vi "Set Manual Volt per Division.vi"(8 "error in (no error)":errorcluster, 9 "V/div":T1, 11 "Oscilloscope in":refnum<class "Oscilloscope.lvclass">) -> (0 "error out":errorcluster, 3 "Oscilloscope out":refnum<class "Oscilloscope.lvclass">)   [LabVIEW 2018, in "Oscilloscope.lvlib" / "Oscilloscope.lvclass"]
uses:
  Oscilloscope.lvclass
  Custom Controls/Volts per Division.ctl
  Custom Controls/Analog Channels.ctl
  Oscilloscope.lvlib
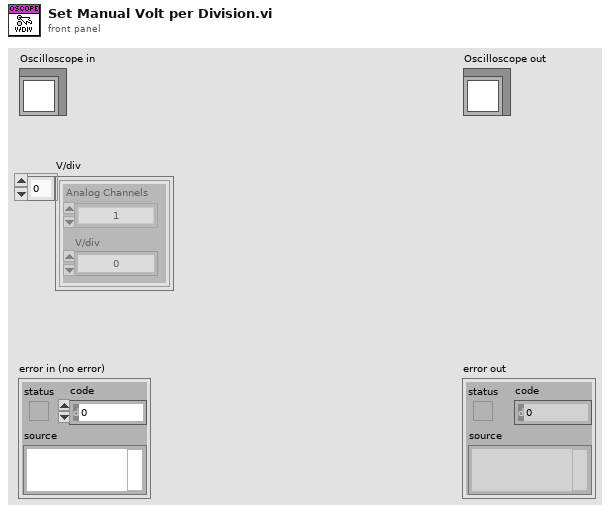
[diagram p1: front panel]
types:
  T1 = typedef "Oscilloscope.lvlib/Volts per Division.ctl" = cluster{"Analog Channels":T2, "V/div":dbl}[]
  T2 = typedef "Oscilloscope.lvlib/Analog Channels.ctl" = enum16{"1", "2", "3", "4", "5", "6", "7", "8", "9", "10", "11", "12", "13", "14", "15", "16"}
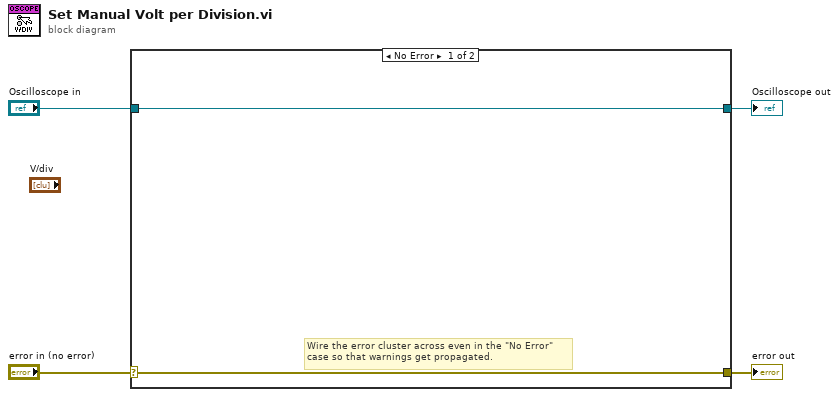
[diagram p0: block diagram]
diagram:
  n1 = case shown="No Error" "error in (no error)" {
    selector: "error in (no error)" -> [w5 w8]
    tunnel: [w5 w8] -> w3
    tunnel: [w6 w7] -> w1
    tunnel: "Oscilloscope in" -> [w6 w7]
    frame No Error {
      # "Wire the error cluster across even in the \"No Error\"\ncase so that warnings get propagated."
    }
    frame Error {
    }
  }
  "error out" <- w3
  "Oscilloscope out" <- w1
